vi "conditional_reset_flexRIO.vi"(4 "reset?":bool, 5 "number in":u16) -> (1 "number out":u16)   [LabVIEW 2010]
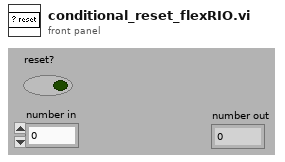
[diagram p1: front panel]
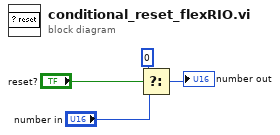
[diagram p0: block diagram]
diagram:
  n1 = Select(t=u16 0, s="reset?", f="number in") -> (s? t:f=→"number out":u16)
